vi "Get Name.vi"(8 "error in (no error)":errorcluster, 11 "Form Configuration in":refnum<class "Form Model Configuration.lvclass">) -> (0 "error out":errorcluster, 2 "Form ID":T1, 3 "Form Configuration out":refnum<class "Form Model Configuration.lvclass">)   [LabVIEW 2020, in "Form Model Configuration.lvlib" / "Form Model Configuration.lvclass"]
uses:
  Form Model Configuration.lvclass
  Autoclose manager/Form ID.ctl
  Form Model Configuration.lvclass/Form Model Configuration.ctl
  Model Panel Logic/Model Panel Logic.lvclass
  Form Server Interfaces.lvlib
  Form Controller/Panel Form Controller.lvclass
  <vilib>/MGI/Panel Manager/Panel/Panel/Panel.lvclass
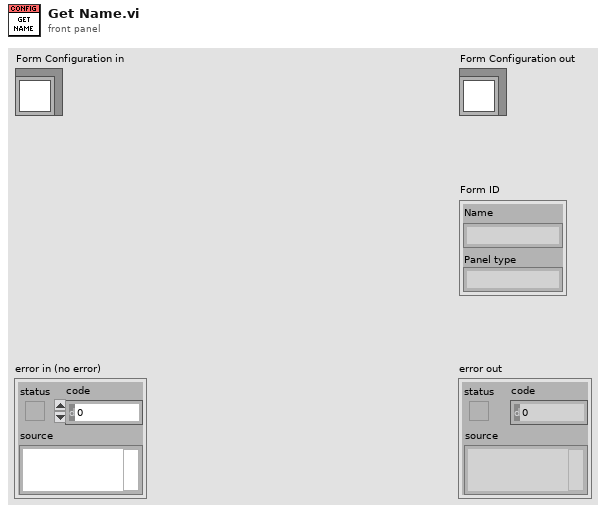
[diagram p1: front panel]
types:
  T1 = typedef "Form Server Interfaces.lvlib/Form ID.ctl" = cluster{"Name":string, "Panel type":string}
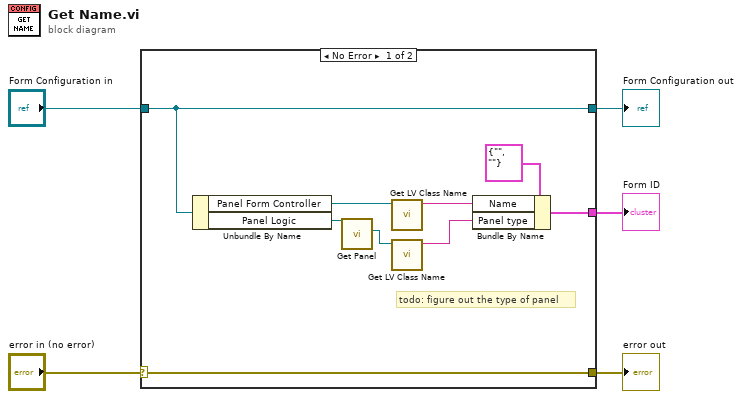
[diagram p0: block diagram]
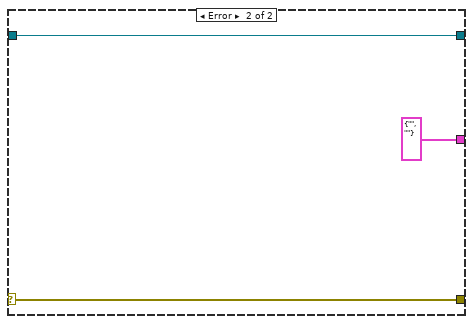
[diagram p2: hidden frame]
diagram:
  n1 = case shown="No Error" "error in (no error)" {
    selector: "error in (no error)" -> [w14 w17]
    tunnel: [w14 w17] -> w4
    tunnel: [w13 w16] -> w2
    tunnel: "Form Configuration in" -> [w13 w16]
    tunnel: [w11 T1 {"Name"="", "Panel type"=""} ("Form ID")] -> w1
    frame No Error {
      # "todo: figure out the type of panel"
      n2 = Unbundle By Name(w13) -> ("Panel Form Controller"=w9:refnum<class "Panel Form Controller.lvclass">, "Panel Logic"=w7:refnum<class "Model Panel Logic.lvclass">)
      n3 = call-dynamic "Get Panel.vi"("Model Panel Logic in"=w7) -> ("Panel"=w6:refnum<class "Panel.lvclass">)  [unwired: 8 in, 2 out]
      n4 = call <vilib>:"Get LV Class Name.vi"("object"=w9) -> ("class name"=w8:string)  [unwired: 9 in, 1 out]
      n5 = call <vilib>:"Get LV Class Name.vi"("object"=w6) -> ("class name"=w10:string)  [unwired: 9 in, 1 out]
      n6 = Bundle By Name(cluster=T1 {"Name"="", "Panel type"=""} ("Form ID"), "Name"=w8, "Panel type"=w10) -> (w11:T1)
    }
    frame Error {
    }
  }
  "error out" <- w4
  "Form Configuration out" <- w2
  "Form ID" <- w1
